vi "Forward Kinematics with DH.vi"(4 "DH Params":cluster{"d_DH":dbl[][], "ty":dbl[][]}, 6 "j4":dbl, 7 "DH Calib?":bool, 8 "j3":dbl, 9 "j2":dbl, 10 "j1":dbl, 11 "armID":i32) -> (1 "XYZ Without Calibration":dbl[](array[numeric]), 2 "XYZ With DH Calibration":dbl[](array[numeric]), 3 "XYZ":dbl[](array[numeric]))   [LabVIEW 2016]
uses:
  <vilib>/Utility/file.llb/Read Delimited Spreadsheet (DBL).vi
panel:
  out "ty":dbl[][](array[numeric])
  out "d_DH":dbl[][](array[numeric])
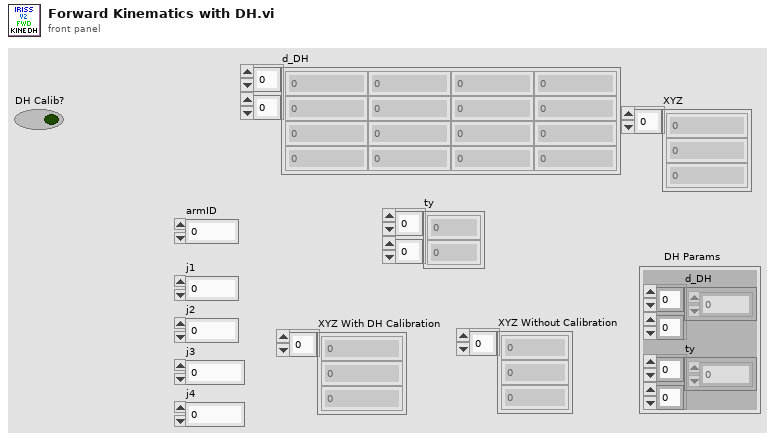
[diagram p1: front panel]
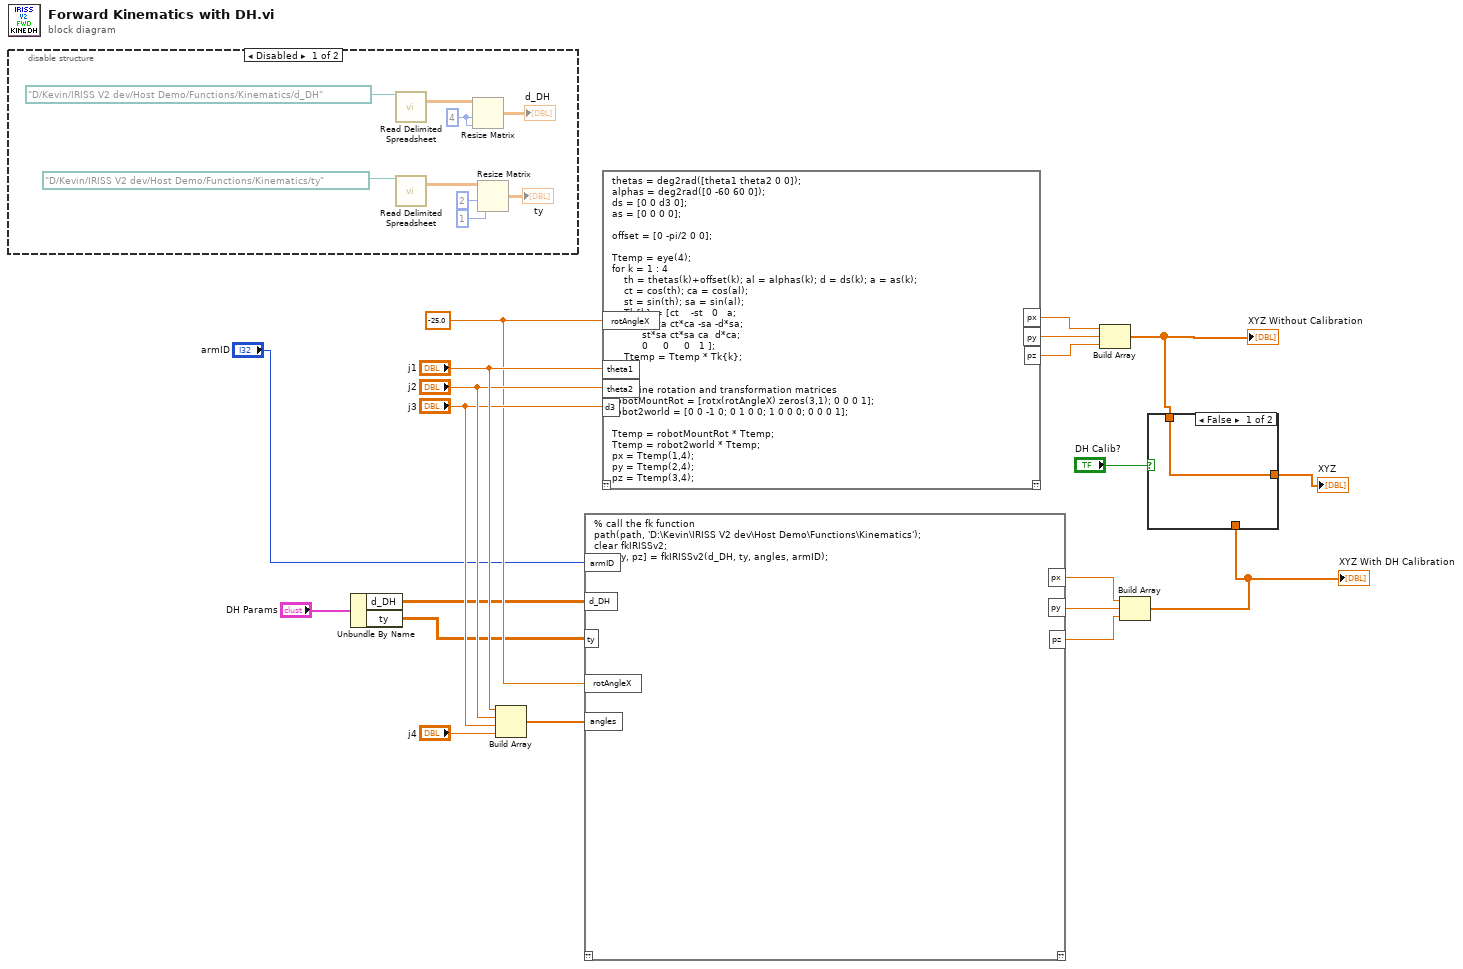
[diagram p0: block diagram]
diagram:
  w13 = -25.0 ("Real")
  n1 = disable-structure shown="Disabled" {
    frame Disabled {
      w27 = 4 ("number of rows")
      n2 = call-poly <vilib>:"Read Delimited Spreadsheet.vi"("file path (dialog if empty)"=path "D:/Kevin/IRISS V2 dev/Host Demo/Functions/Kinematics/d_DH" ("file path (use dialog)")) -> ("all rows"=w28:dbl[][])  [unwired: 9 in, 5 out]
      n3 = call-poly <vilib>:"Read Delimited Spreadsheet.vi"("file path (dialog if empty)"=path "D:/Kevin/IRISS V2 dev/Host Demo/Functions/Kinematics/ty" ("file path (use dialog)")) -> ("all rows"=w25:dbl[][])  [unwired: 9 in, 5 out]
      n4 = Resize Matrix(1:w27, 2:w27, 4:w28) -> (0:→"d_DH":dbl[][])
      n5 = Resize Matrix(1:1 ("number of columns"), 2:2 ("number of rows"), 4:w25) -> (0:→"ty":dbl[][])
    }
    frame Enabled {
    }
  }
  n6 = Unbundle By Name("DH Params") -> ("d_DH"=w7:dbl[][], "ty"=w6:dbl[][])
  n7 = Build Array("j1", "j2", "j3", "j4") -> (w14:dbl[])
  n8 = script code="% call the fk function\npath(path, 'D:\\Kevin\\IRISS V2 dev\\Host Demo\\Functions\\Kinematics');\nclear fkIRISSv2;\n[px, py, pz] = fkIRISSv2(d_DH, ty, angles, armID);"("angles"=w14, "rotAngleX"=w13, "d_DH"=w7, "ty"=w6, "armID"="armID") -> ("px"=w11:dbl, "py"=w12:dbl, "pz"=w10:dbl)  [unwired: 1 in, 1 out]
  n9 = script code="thetas = deg2rad([theta1 theta2 0 0]);\nalphas = deg2rad([0 -60 60 0]);\nds = [0 0 d3 0];\nas = [0 0 0 0];\n\noffset = [0 -pi/2 0 0];\n\nTtemp = eye(4);\nfor k = 1 : 4\n    th = thetas(k)+offset(k); al = alphas(k); d = ds(k); a = as(k);\n    ct = cos(th); ca = cos(al);\n    st = sin(th); sa = sin(al);\n    Tk{k} = [ct    -st   0   a;\n          st*ca ct*ca -sa -d*sa;\n          st*sa ct*sa ca  d*ca;\n          0     0     0   1 ];\n    Ttemp = Ttemp * Tk{k};\nend\n\n% define rotation and transformation matrices\nrobotMountRot = [rotx(rotAngleX) zeros(3,1); 0 0 0 1];\nrobot2world = [0 0 -1 0; 0 1 0 0; 1 0 0 0; 0 0 0 1];\n\nTtemp = robotMountRot * Ttemp;\nTtemp = robot2world * Ttemp;\npx = Ttemp(1,4);\npy = Ttemp(2,4);\npz = Ttemp(3,4);"("theta1"="j1", "theta2"="j2", "d3"="j3", "rotAngleX"=w13) -> ("px"=w20:dbl, "py"=w19:dbl, "pz"=w18:dbl)  [unwired: 1 in, 1 out]
  n10 = Build Array(w20, w19, w18) -> (w2:dbl[])
  "XYZ Without Calibration" <- w2
  n11 = Build Array(w11, w12, w10) -> (w3:dbl[])
  "XYZ With DH Calibration" <- w3
  n12 = case shown="False" "DH Calib?" {
    tunnel: w3 -> [_ w31]
    tunnel: w2 -> [w30 _]
    tunnel: [w30 w31] -> w1
    frame False {
    }
    frame True {
    }
  }
  "XYZ" <- w1
